vi "CTRE_ErrorHandle.vi"(8 "error in":errorcluster, 10 "origin":string, 11 "code":i32) -> (0 "error out":errorcluster)   [LabVIEW 2017]
uses:
  <vilib>/Utility/error.llb/whitespace.ctl
  Public/Documents/Cross The Road Electronics/Phoenix-LabVIEW/Controls/DriverLib.ctl
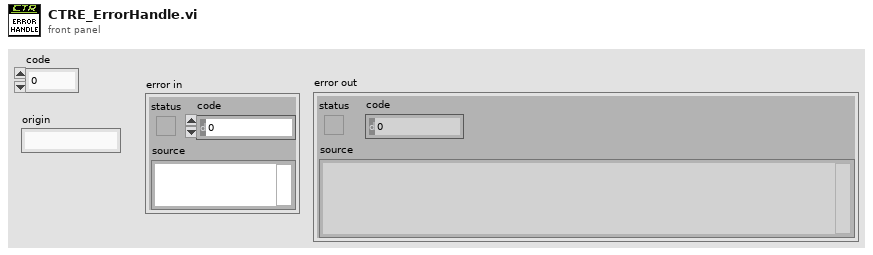
[diagram p1: front panel]
types:
  T1 = typedef "DriverLib.ctl" = path
  T2 = typedef "whitespace.ctl" = u16
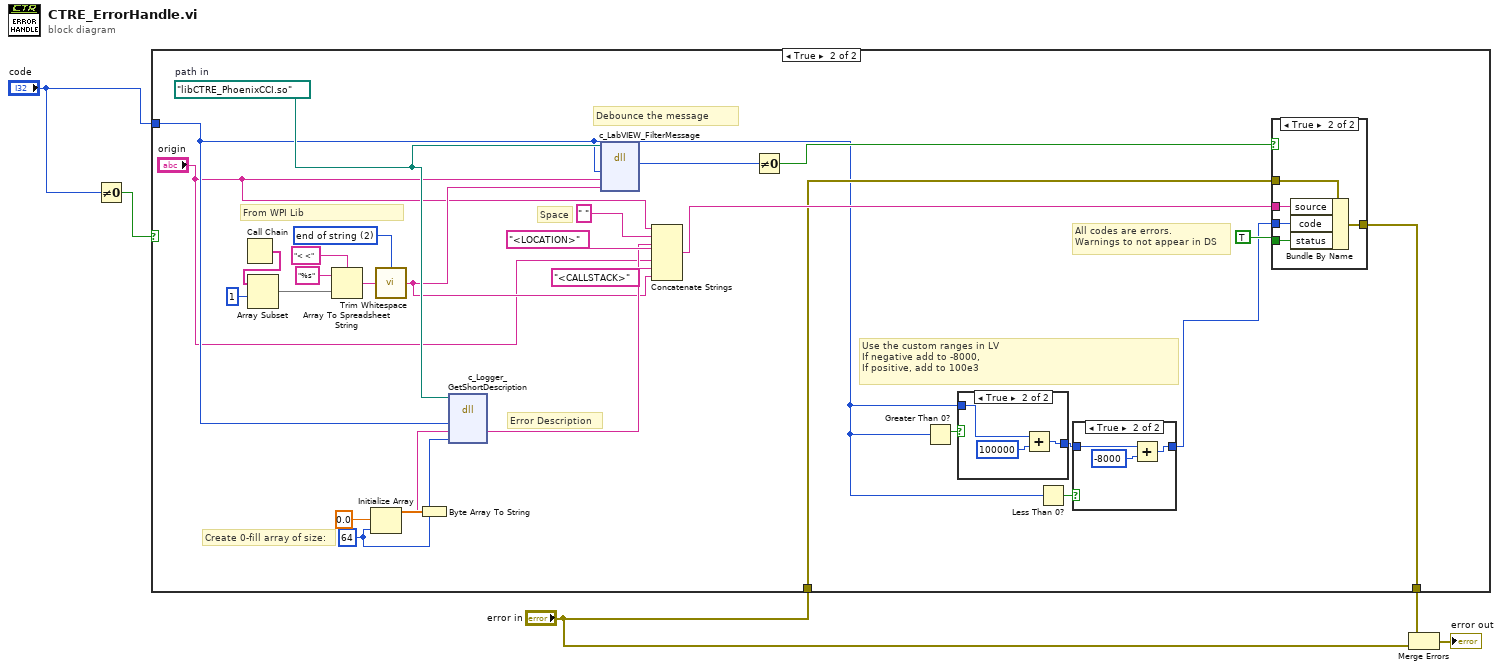
[diagram p0: block diagram]
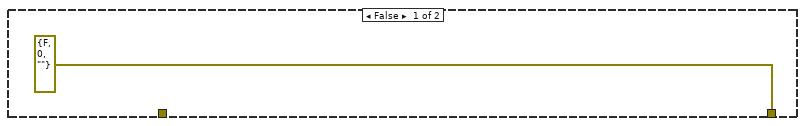
[diagram p2: hidden frame]
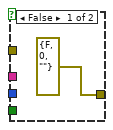
[diagram p5: hidden frame]
diagram:
  n1 = Not Equal To 0?(x="code") -> (x != 0?=w4:bool)
  n2 = case shown="True" w4 {
    tunnel: "error in" -> [_ w17]
    tunnel: "code" -> [_ w11]
    tunnel: [errorcluster {"status"=FALSE, "code"=0, "source"=""} ("error in") w18] -> w1
    frame False {
    }
    frame True {
      w24 = 64 ("dimension size")
      w16 = T1 path "libCTRE_PhoenixCCI.so"  # path in
      w32 = T2 2 items=["both", "start of string", "end of string"] ("location (both)")
      # "Space"
      # "Debounce the message"
      # "Use the custom ranges in LV\nIf negative add to -8000,\nIf positive, add to 100e3"
      # "All codes are errors.\nWarnings to not appear in DS"
      # "Error Description"
      # "Create 0-fill array of size:"
      # "From WPI Lib"
      n3 = Call Chain() -> (call chain=w29:string[])
      n4 = Array Subset(array=w29, index=1) -> (w30:string[])  [unwired: 1 in]
      n5 = Array To Spreadsheet String(delimiter (Tab)="< <", array=w30, 3:"%s" ("format string")) -> (spreadsheet string=w33:string)
      n6 = Initialize Array(0.0 ("element"), w24) -> (w26:dbl[])
      n7 = call <vilib>:"Trim Whitespace.vi"("string"=w33, "location (both)"=w32) -> ("trimmed string"=w9:string)
      n8 = Byte Array To String(unsigned byte array=w26) -> (string=w25:string)
      n9 = dll-call lib="?" fn="c_Logger_GetShortDescription"(path in=w16, "CTRCode"=w11, "toFill"=w25, "capacity"=w24) -> ("toFill"=w10:string)  [unwired: 5 in, 2 out]
      n10 = dll-call lib="?" fn="c_LabVIEW_FilterMessage"(path in=w16, "CTRCode"=w11, "origin"="origin", "stacktrace"=w9) -> ("return type"=w22:i32)  [unwired: 5 in, 2 out]
      n11 = Concatenate Strings("origin", " " ("string"), w10, "<LOCATION>" ("string"), "origin", "<CALLSTACK>" ("string"), w9) -> (w20:string)
      n12 = Not Equal To 0?(x=w22) -> (x != 0?=w21:bool)
      n13 = Greater Than 0?(x=w11) -> (x > 0?=w15:bool)
      n14 = case shown="True" w15 {
        tunnel: w11 -> [w40 w43]
        tunnel: [w40 w41] -> w13
        frame False {
        }
        frame True {
          n15 = Add(x=w43, y=100000) -> (x+y=w41:i32)
        }
      }
      n16 = Less Than 0?(x=w11) -> (x < 0?=w14:bool)
      n17 = case shown="True" w14 {
        tunnel: w13 -> [w36 w38]
        tunnel: [w36 w39] -> w12
        frame False {
        }
        frame True {
          n18 = Add(x=w38, y=-8000) -> (x+y=w39:i32)
        }
      }
      n19 = case shown="True" w21 {
        tunnel: w17 -> [_ w49]
        tunnel: w20 -> [_ w48]
        tunnel: w12 -> [_ w47]
        tunnel: TRUE ("status") -> [_ w46]
        tunnel: [errorcluster {"status"=FALSE, "code"=0, "source"=""} ("error in") w45] -> w18
        frame False {
        }
        frame True {
          n20 = Bundle By Name(cluster=w49, "source"=w48, "code"=w47, "status"=w46) -> (w45:errorcluster)
        }
      }
    }
  }
  n21 = Merge Errors(w1, "error in") -> (→"error out":errorcluster)
